vi "Get Data.vi"(8 "error in":errorcluster, 11 "nCRD in":refnum<class "gCRD.lvclass">) -> (0 "error out":errorcluster, 3 "nCRD out":refnum<class "gCRD.lvclass">)   [LabVIEW 2017, in "gCRDS.lvlib" / "gCRD.lvclass"]
doc: "Retrieve the data from the given cards. Set the <B>goodData</B> flag to True and log any errors that will be handled down the line. If there is an error associated with the collection of the data, the <B>goodData</B> flag will be set to false when the logged errors are handled.\nThe ringdown traces recorded in the <B>HF AI</B> task are divided up into a m x n matrix where:\n * m = YAG pulse rate\n * n = YAG duty cycle * HF AI Sampling Rate / YAG Pulse Rate"
uses:
  gCRD.lvclass
  C:/Program Files (x86)/National Instruments/LabVIEW 2017/vi.lib/MSR Consulting, LLC/General Reuse/CRDS/Main/CRDS.lvclass
  C:/Program Files (x86)/National Instruments/LabVIEW 2017/vi.lib/MSR Consulting, LLC/General Reuse/Instrument/Instrument.lvclass
  gCRD.lvclass/gCRD.ctl
  <vilib>/MSR Consulting, LLC/General Reuse/Instrument/state.ctl
  <vilib>/MSR Consulting, LLC/General Reuse/CRDS/Main/CRDS.lvclass/CRDS.ctl
  <vilib>/MSR Consulting, LLC/General Reuse/Instrument/Instrument.lvclass/Instrument.ctl
  <vilib>/MSR Consulting, LLC/General Reuse/CRDS/Cell/CRDS Cell.lvclass/CRDS Cell.ctl
  <vilib>/MSR Consulting, LLC/General Reuse/CRDS/Cell/Write Laser Data.vi
  <vilib>/MSR Consulting, LLC/General Reuse/CRDS/Main/Write NumCoadd.vi
  <vilib>/MSR Consulting, LLC/General Reuse/Instrument/Read Data.vi
  <vilib>/MSR Consulting, LLC/General Reuse/Instrument/Read Log Session.vi
  <vilib>/MSR Consulting, LLC/General Reuse/Instrument/Write Data.vi
  <vilib>/MSR Consulting, LLC/General Reuse/Instrument/Write Data OK_.vi
  <vilib>/Utility/error.llb/Error Cluster From Error Code.vi
  <vilib>/rvi/errors/niLvFpgaAdjustHostInterfaceError.vi
  <vilib>/MSR Consulting, LLC/General Reuse/Data/Write measTime.vi
  <vilib>/MSR Consulting, LLC/General Reuse/CRDS/Main/Read Cells.vi
  <vilib>/MSR Consulting, LLC/General Reuse/CRDS/Main/Write Cells.vi
  <vilib>/MSR Consulting, LLC/General Reuse/Data/Data.lvclass
  <vilib>/MSR Consulting, LLC/General Reuse/Session APIs/_Session Fwk/Session - Root.lvclass
  <vilib>/rvi/interface/nirviMethod/nirviMethod.xnode
  FPGA Ref.ctl
  FPGA Bitfiles/server.lvbitx
  <vilib>/MSR Consulting, LLC/General Reuse/CRDS/Cell/CRDS Cell.lvclass
  <vilib>/MSR Consulting, LLC/General Reuse/CRDS/Main/CRDS.lvclass
  <vilib>/MSR Consulting, LLC/General Reuse/Instrument/Instrument.lvclass
  <vilib>/MSR Consulting, LLC/General Reuse/Session APIs/Session Log/System Log.lvclass
  <vilib>/FPGAPlugInAG/cRIO-9081/niLvFpga_ReadFifo_cRIO-9081.vi
  <vilib>/rvi/errors/niLvFpgaMergeErrorWithErrorCode.vi
panel:
  in  "index (row) 2":i32
  out "Discontinuity Detected 2":bool
  out "Discontinuity Detected":bool
  out "wvg2":i16[](graph)
  out "wvg":i16[](graph)
  out "eRemaining":u32
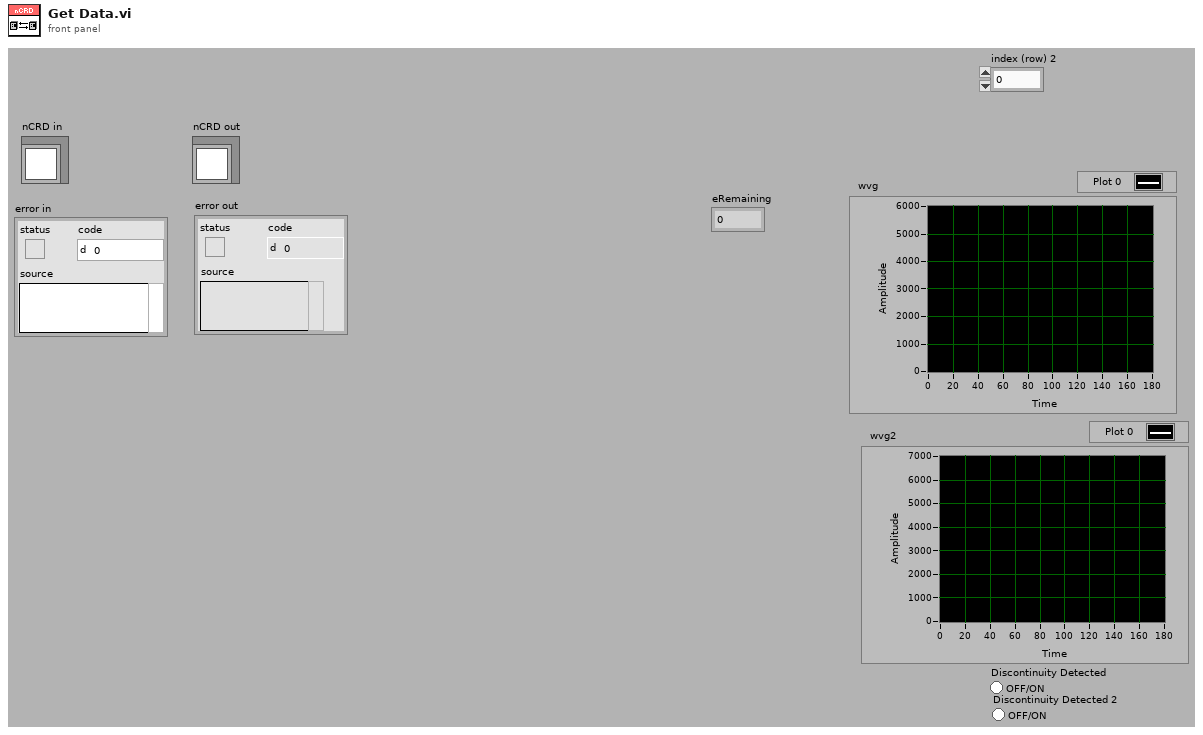
[diagram p1: front panel]
types:
  T1 = typedef "Instrument.lvclass/state.ctl" = enum8{"Configure", "Acquire", "Wait", "Quit", "Handle Error", "NOOP"}
  T2 = typedef "FPGA Ref.ctl" = refnum<k20>
  T3 = typedef "Session - Root.lvclass/Session Handle.ctl" = refnum<data-value>
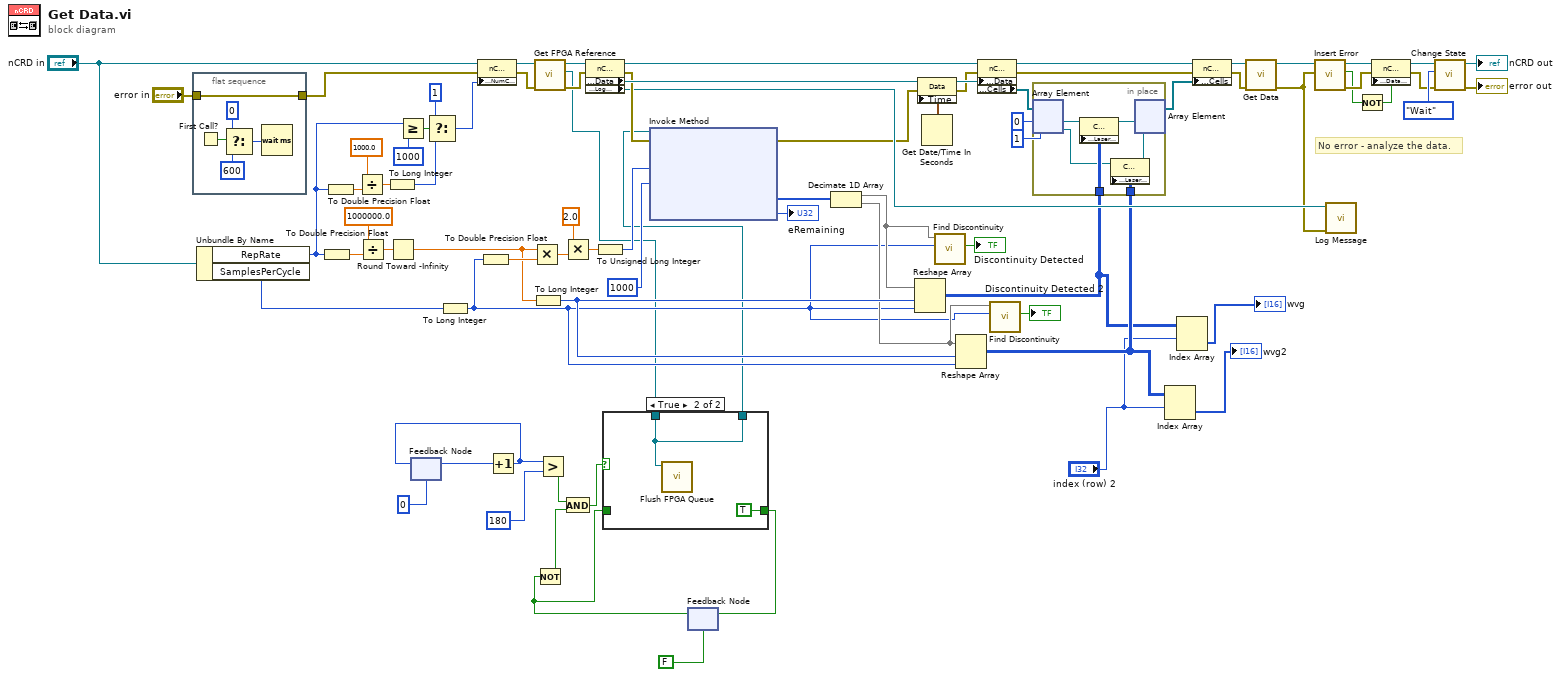
[diagram p0: block diagram]
diagram:
  # "No error - analyze the data."
  n1 = flat-sequence {
    tunnel: "error in" -> [w84]
    tunnel: [w84] -> w35
    frame #0 {
      n2 = First Call?() -> (First Call?: T/F=w83:bool)
      n3 = Select(t=u32 0, s=w83, f=u32 600) -> (s? t:f=w80:u32)
      n4 = Wait (ms)(milliseconds to wait=w80) -> ()  [unwired: 1 out]
    }
  }
  n5 = Unbundle By Name("nCRD in") -> ("RepRate"=w27:u16, "SamplesPerCycle"=w74:u16)
  n6 = To Double Precision Float(number=w27) -> (double precision float=w54:dbl)
  n7 = To Double Precision Float(number=w27) -> (double precision float=w26:dbl)
  n8 = Divide(x=1000.0 ("y"), y=w26) -> (x/y=w25:dbl)
  n9 = Divide(x=1000000.0, y=w54) -> (x/y=w53:dbl)
  n10 = To Long Integer(number=w25) -> (32bit integer=w24:i32)
  n11 = Round Toward -Infinity(1:w53) -> (0:w43:dbl)
  n12 = Greater Or Equal?(x=w27, y=u16 1000) -> (x >= y?=w31:bool)
  n13 = feedback #1(0) -> (w17:i32)
  n14 = Select(t=1 ("NumCoadd"), s=w31, f=w24) -> (s? t:f=w23:i32)
  n15 = To Long Integer(number=w74) -> (32bit integer=w19:i32)
  n16 = property class="nCRD"(reference="nCRD in", error in=w35, "Data Access:NumCoadd"=w23) -> (reference out=w34:refnum<class "gCRD.lvclass">, error out=w33:errorcluster)
  n17 = To Double Precision Float(number=w19) -> (double precision float=w52:dbl)
  n18 = Increment(x=w17) -> (x+1=w15:i32)
  n19 = feedback-in #1(w15) -> ()
  n20 = Multiply(x=w43, y=w52) -> (x*y=w59:dbl)
  n21 = To Long Integer(number=w43) -> (32bit integer=w42:i32)
  n22 = call "Get FPGA Reference.vi"("error in"=w33, "nCRD in"=w34) -> ("error out"=w41:errorcluster, "FPGA Ref"=w11:T2, "nCRD out"=w57:refnum<class "gCRD.lvclass">)  [unwired: 7 in]
  n23 = Greater?(x=w15, y=180) -> (0:w12:bool)
  n24 = Multiply(x=2.0, y=w59) -> (x*y=w58:dbl)
  n25 = property class="nCRD"(reference=w57, error in=w41) -> (reference out=w70:refnum<class "gCRD.lvclass">, error out=w56:errorcluster, "Accessors:Data"=w69:refnum<class "Data.lvclass">, "Accessors:Log Session"=w55:T3)
  n26 = To Unsigned Long Integer(number=w58) -> (unsigned 32bit integer=w50:u32)
  n27 = feedback #2(FALSE) -> (w7:bool)
  n28 = Not(x=w7) -> (.not. x?=w8:bool)
  n29 = And(x=w12, y=w8) -> (x .and. y?=w13:bool)
  n30 = case shown="True" w13 {
    tunnel: w11 -> [w86 w88]
    tunnel: [w86 w88] -> w10
    tunnel: w7 -> [w85 _]
    tunnel: [w85 TRUE] -> w6
    frame False {
    }
    frame True {
      n31 = call "Flush FPGA Queue.vi"("Refnum in"=w88) -> ()  [unwired: 10 in, 1 out]
    }
  }
  n32 = xnode "Invoke Method"("FPGA VI Reference In"=w10, "error in"=w56, "Number of Elements"=w50, "Timeout (ms)"=1000) -> ("error out"=w51:errorcluster, "Data"=w46:i16[], "Elements Remaining"=→"eRemaining":u32)  [unwired: 1 out]
  n33 = feedback-in #2(w6) -> ()
  n34 = Decimate 1D Array(w46) -> (w22:i16[], w20:i16[])
  n35 = Reshape Array(w22, w42, w19) -> (w3:i16[][])
  n36 = Get Date/Time In Seconds() -> (seconds since 1Jan1904=w68:timestamp)
  n37 = property class="Data"(reference=w69, error in=w51, "Time"=w68) -> (reference out=w67:refnum<class "Data.lvclass">, error out=w66:errorcluster)
  n38 = call <vilib>:"Find Discontinuity.vi"("Single Record"=w19, "Data"=w22) -> ("Discontinuity Detected"=→"Discontinuity Detected":bool)  [unwired: 8 in, 1 out]
  n39 = Reshape Array(w20, w42, w19) -> (w5:i16[][])
  n40 = property class="nCRD"(reference=w70, error in=w66, "Accessors:Data"=w67) -> (reference out=w65:refnum<class "gCRD.lvclass">, error out=w61:errorcluster, "Data Access:Cells"=w64:refnum<class "CRDS Cell.lvclass">[])
  n41 = call <vilib>:"Find Discontinuity.vi"("Single Record"=w19, "Data"=w20) -> ("Discontinuity Detected"=→"Discontinuity Detected 2":bool)  [unwired: 8 in, 1 out]
  n42 = in-place {
    in-place-border: w3 -> [w93]
    in-place-border: w5 -> [w89]
    n43 = in-place-array #3(w64, 0, 1) -> (w94:refnum<class "CRDS Cell.lvclass">, w91:refnum<class "CRDS Cell.lvclass">)
    n44 = property class="CRDS Cell"(reference=w94, "Accessors:Laser Data"=w93) -> (reference out=w92:refnum<class "CRDS Cell.lvclass">)  [unwired: 1 in, 1 out]
    n45 = property class="CRDS Cell"(reference=w91, "Accessors:Laser Data"=w89) -> (reference out=w90:refnum<class "CRDS Cell.lvclass">)  [unwired: 1 in, 1 out]
    n46 = in-place-array #3(w92, w90) -> (w62:refnum<class "CRDS Cell.lvclass">[])  [unwired: 2 out]
  }
  n47 = Index Array(array=w5, index (row)="index (row) 2") -> (element=→"wvg2":i16[])  [unwired: 1 in]
  n48 = Index Array(array=w3, index (row)="index (row) 2") -> (element=→"wvg":i16[])  [unwired: 1 in]
  n49 = property class="nCRD"(reference=w65, error in=w61, "Data Access:Cells"=w62) -> (reference out=w40:refnum<class "gCRD.lvclass">, error out=w37:errorcluster)
  n50 = call-parent "Get Data.vi"("error in"=w37, "CRDS in"=w40) -> ("error out"=w38:errorcluster, "CRDS out"=w39:refnum<class "gCRD.lvclass">)  [unwired: 8 in]
  n51 = call <vilib>:"Insert Error.vi"("err"=w38, "Instrument in"=w39) -> ("error out"=w72:errorcluster, "error?"=w71:bool, "Instrument out"=w73:refnum<class "gCRD.lvclass">)  [unwired: 7 in]
  n52 = call <vilib>:"Log Message.vi"("error in"=w38, "session in"=w55) -> ()  [unwired: 8 in, 2 out]
  n53 = Not(x=w71) -> (.not. x?=w47:bool)
  n54 = property class="nCRD"(reference=w73, error in=w72, "Accessors:Data OK_"=w47) -> (reference out=w76:refnum<class "gCRD.lvclass">, error out=w75:errorcluster)
  n55 = call <vilib>:"Change State.vi"("error in"=w75, "instr state"=state."Wait", "Instrument in"=w76) -> ("error out"=→"error out":errorcluster, "Instrument out"=→"nCRD out":refnum<class "gCRD.lvclass">)  [unwired: 7 in]
